vi "Set.vi"(7 "Binding":refnum<class "Binding.lvclass">, 8 "error in (no error)":errorcluster, 10 "Value":variant, 11 "Class in":refnum<class>) -> (0 "error out":errorcluster, 3 "Class out":refnum<class>)   [LabVIEW 2020, in "PropertyBinder.lvlib" / "Binding.lvclass"]
uses:
  Binding.lvclass
  Binding.lvclass/Binding.ctl
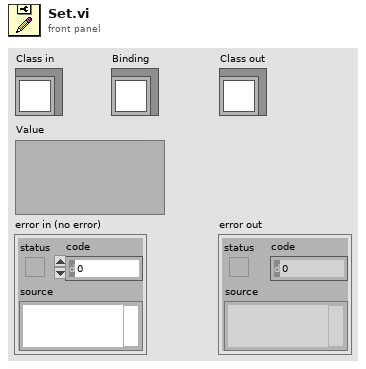
[diagram p1: front panel]
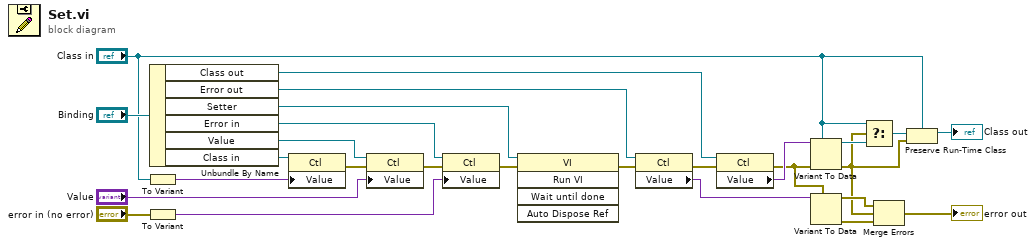
[diagram p0: block diagram]
diagram:
  n1 = To Variant(anything="Class in") -> (Variant=w16:variant)
  n2 = To Variant(anything="error in (no error)") -> (Variant=w11:variant)
  n3 = Unbundle By Name("Binding") -> ("Class out"=w1:refnum<vi>, "Error out"=w7:refnum<vi>, "Setter"=w18:refnum<vi>, "Error in"=w12:refnum<vi>, "Value"=w14:refnum<vi>, "Class in"=w17:refnum<vi>)
  n4 = property class="Ctl"(reference=w17, "Value"=w16) -> (error out=w15:errorcluster)  [unwired: 1 in, 1 out]
  n5 = property class="Ctl"(reference=w14, error in=w15, "Value"="Value") -> (error out=w13:errorcluster)  [unwired: 1 out]
  n6 = property class="Ctl"(reference=w12, error in=w13, "Value"=w11) -> (error out=w10:errorcluster)  [unwired: 1 out]
  n7 = invoke class="VI" method="Run VI"(reference=w18, error in=w10) -> (error out=w9:errorcluster)  [unwired: 3 in, 4 out]
  n8 = property class="Ctl"(reference=w7, error in=w9) -> (error out=w8:errorcluster, "Value"=w6:variant)  [unwired: 1 out]
  n9 = property class="Ctl"(reference=w1, error in=w8) -> (error out=w2:errorcluster, "Value"=w3:variant)  [unwired: 1 out]
  n10 = Variant To Data(error in=w2, type="Class in", Variant=w3) -> (data=w21:refnum<class>, error out=w4:errorcluster)
  n11 = Variant To Data(type=w2, Variant=w6) -> (data=w5:errorcluster, error out=w24:errorcluster)  [unwired: 1 in]
  n12 = Select(t="Class in", s=w4, f=w21) -> (s? t:f=w19:refnum<class>)
  n13 = Merge Errors(w5, w4, w24) -> (→"error out":errorcluster)
  n14 = Preserve Run-Time Class(object in=w19, error in=w4, 2:"Class in") -> (object out=→"Class out":refnum<class>)  [unwired: 1 out]
